vi "Begin.vi"(11 "Image Size":T1=enum."160x120") -> (0 "error out":errorcluster)   [LabVIEW 2012]
doc: "Called before other user functions, this VI is expected to open initial I/O refnums, load in file data, and do all program initialization. Notice that the <B>error out</B> terminal is simply used for data flow. Wiring it to other structures or subVIs ensures that this VI runs first."
uses:
  <vilib>/Rock Robotics/WPI/Camera/WPI_CameraImageSize.ctl
  <vilib>/Rock Robotics/WPI/Camera/WPI_CameraWhite Balance Values.ctl
  <vilib>/Rock Robotics/WPI/Camera/WPI_CameraExposure Values.ctl
  <vilib>/Rock Robotics/WPI/Camera/WPI_CameraFrameRate.ctl
  <vilib>/Rock Robotics/WPI/DriverStation/WPI_DriverStationRobotMode2.ctl
  <vilib>/Rock Robotics/WPI/Joystick/WPI_JoystickDeviceEnum.ctl
  <vilib>/Rock Robotics/SystemInterfaces/DIO/FPGA_DIORelayChannel.ctl
  <vilib>/Rock Robotics/WPI/Relay/WPI_RelayDirection.ctl
  <vilib>/Rock Robotics/SystemInterfaces/DIO/FPGA_DIOPWMChannel.ctl
  <vilib>/Rock Robotics/SystemInterfaces/DIO/FPGA_DIOChannel.ctl
  <vilib>/Rock Robotics/WPI/Solenoid/WPI_SolenoidChannel.ctl
  <vilib>/Rock Robotics/WPI/Relay/WPI_RelayValue.ctl
  <vilib>/Rock Robotics/WPI/SafetyOutput/WPI_SafetyOutputConfigMenu.ctl
  Robot Global Data.vi
  <vilib>/Rock Robotics/WPI/Solenoid/WPI_SolenoidOpenSingle.vi
  <vilib>/Rock Robotics/WPI/MotorControl/WPI_MotorControlOpen Victor.vi
  <vilib>/Rock Robotics/WPI/RobotDrive/WPI_RobotDriveOpen2MotorWithTalon.vi
  <vilib>/Rock Robotics/WPI/Compressor/WPI_CompressorGetSetRefNum.vi
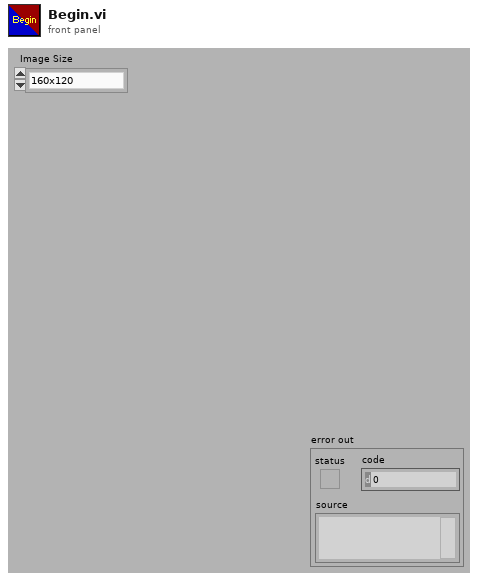
[diagram p1: front panel]
types:
  T1 = typedef "WPI_CameraImageSize.ctl" = enum16{"640x480", "320x240", "160x120"}
  T2 = typedef "FPGA_DIOChannel.ctl" = enum8{"DIO 1", "DIO 2", "DIO 3", "DIO 4", "DIO 5", "DIO 6", "DIO 7", "DIO 8", "DIO 9", "DIO 10", "DIO 11", "DIO 12", "DIO 13", "DIO 14", "Invalid"}
  T3 = typedef "WPI_JoystickDeviceEnum.ctl" = enum16{"USB 1", "USB 2", "USB 3", "USB 4", "Kinect 1", "Kinect 2"}
  T4 = typedef "WPI_SafetyOutputConfigMenu.ctl" = enum16{"Enable", "Disable"}
  T5 = typedef "WPI_SolenoidChannel.ctl" = enum8{"Solenoid 1", "Solenoid 2", "Solenoid 3", "Solenoid 4", "Solenoid 5", "Solenoid 6", "Solenoid 7", "Solenoid 8", "Invalid"}
  T6 = typedef "FPGA_DIOPWMChannel.ctl" = enum8{"PWM 1", "PWM 2", "PWM 3", "PWM 4", "PWM 5", "PWM 6", "PWM 7", "PWM 8", "PWM 9", "PWM 10", "Invalid"}
  T7 = typedef "WPI_RelayValue.ctl" = enum16{"Off", "On", "Forward", "Reverse"}
  T8 = typedef "FPGA_DIORelayChannel.ctl" = enum8{"Relay 1", "Relay 2", "Relay 3", "Relay 4", "Relay 5", "Relay 6", "Relay 7", "Relay 8", "Invalid"}
  T9 = typedef "WPI_RelayDirection.ctl" = enum16{"Both directions", "Forward only", "Reverse only"}
  T10 = typedef "WPI_DriverStationRobotMode2.ctl" = enum16{"Autonomous Disabled", "Autonomous Enabled", "Teleop Disabled", "Teleop Enabled", "Timeout", "Finish", "Test Disabled", "Test Enabled"}
  T11 = typedef "WPI_CameraFrameRate.ctl" = u32
  T12 = typedef "WPI_CameraExposure Values.ctl" = enum16{"Auto", "Flicker-free 50 Hz", "Flicker-free 60 Hz", "Hold current"}
  T13 = typedef "WPI_CameraWhite Balance Values.ctl" = enum16{"Auto", "Fixed indoor", "Fixed outdoor 1", "Fixed outdoor 2", "Fixed fluorescent 1", "Fixed fluorescent 2", "Hold current"}
  T14 = typedef "WPI_MotorControlDeviceRef.ctl" = cluster{"DeviceStatus":errorcluster, "Type":enum16{"PWM", "CAN"}, "PWM":cluster{"Digital Module":T15, "PWM Channel":T6, "DeadBand":T16}, "CAN":cluster{"Device Number":u8, "Control Mode":T17, "Semaphore":T18, "Max Vout":dbl}, "Invert":bool, "TransformRef":T19, "InvTransformRef":T19}
  T15 = typedef "FPGA_TypedefDigitalModule.ctl" = enum16{"Digital Module 1", "Digital Module 2"}
  T16 = typedef "WPI_PWMDeadband.ctl" = cluster{"Name":string, "maxPositivePwm":i32, "minPositivePwm":i32, "centerPwm":i32, "maxNegativePwm":i32, "minNegativePwm":i32, "angularRange":u16}
  T17 = typedef "WPI_CANJaguar_ControlMode.ctl" = enum8{"Percent VBus", "Current", "Speed", "Position", "Voltage"}
  T18 = typedef "Semaphore RefNum" = refnum<k1>
  T19 = typedef "WPI_PWMTransform_ConPane.ctl" = refnum<vi>
  T20 = typedef "WPI_ServoDeviceRef.ctl" = cluster{"DeviceStatus":errorcluster, "Digital Module":T15, "PWM Channel":T6, "DeadBand":T16}
  T21 = typedef "WPI_JoystickDevRef.ctl" = cluster{"Device":T3}
  T22 = typedef "WPI_CameraDevRef.ctl" = cluster{"Camera Address":string, "CameraStatus":errorcluster, "Acquire Image Notifier":refnum<notifier>}
  T23 = typedef "WPI_RobotDriveDevRef.ctl" = cluster{"DevStatus":errorcluster, "Motors[]":T14[], "Square Inputs":bool, "Max Output":dbl, "Isochronous":bool}
  T24 = typedef "WPI_RelayDevRef.ctl" = cluster{"DevStatus":errorcluster, "Relay Channel":T8, "Digital Module":T15, "Relay Direction":T9}
  T25 = typedef "WPI_SolenoidDevRef.ctl" = cluster{"DevStatus":errorcluster, "Solenoid Module":T26, "Forward Solenoid Channel":T5, "Reverse Solenoid Channel":T5}
  T26 = typedef "FPGA_TypedefSolenoidModule.ctl" = enum16{"Solenoid Module 1", "Solenoid Module 2"}
  T27 = typedef "WPI_DigitalInputDevRef.ctl" = cluster{"DevStatus":errorcluster, "DIO Channel":T2, "Digital Module":T15}
  T28 = typedef "WPI_CompressorDevRef.ctl" = cluster{"DevStatus":errorcluster, "DigitalInputDevRef":T27, "RelayDevRef":T24}
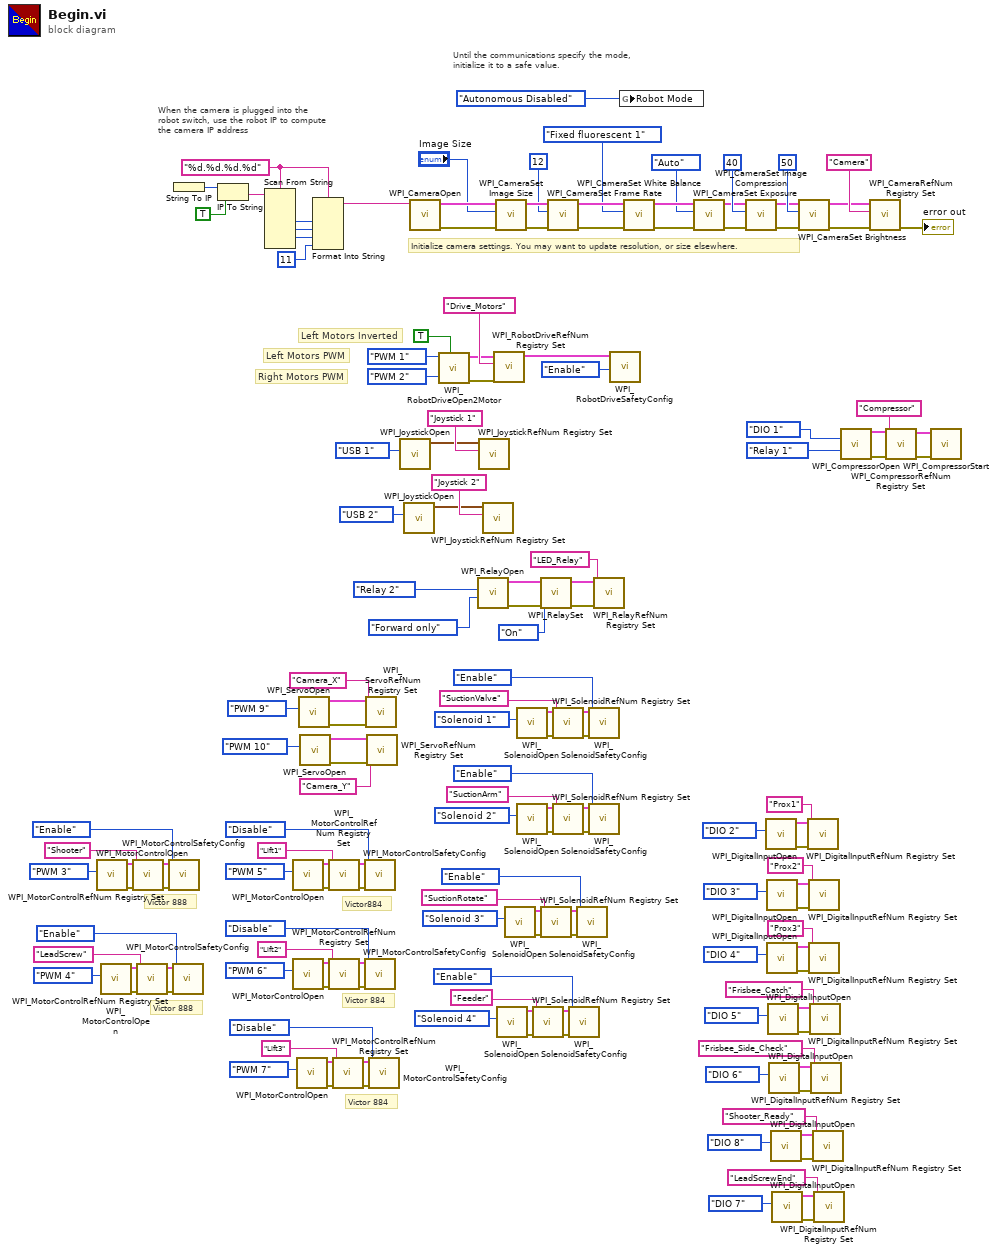
[diagram p0: block diagram]
diagram:
  w131 = "%d.%d.%d.%d" ("format string")
  # "Victor884"
  # "Victor 884"
  # "Victor 884"
  # "Victor 888"
  # "Victor 888"
  # "Right Motors PWM"
  # "Left Motors PWM"
  # "Left Motors Inverted"
  # "Until the communications specify the mode,\ninitialize it to a safe value."
  # "When the camera is plugged into the\nrobot switch, use the robot IP to compute\nthe camera IP address"
  # "Initialize camera settings. You may want to update resolution, or size elsewhere."
  n1 = call-poly <vilib>:"WPI_MotorControlOpen.vi"("PWM Channel"=FPGA_DIOPWMChannel."PWM 3") -> ("error out"=w37:errorcluster, "MotorControlDeviceRef"=w38:T14)  [unwired: 9 in]
  n2 = call-poly <vilib>:"WPI_MotorControlOpen.vi"("PWM Channel"=FPGA_DIOPWMChannel."PWM 4") -> ("error out"=w93:errorcluster, "MotorControlDeviceRef"=w94:T14)  [unwired: 9 in]
  n3 = call <vilib>:"WPI_MotorControlRefNum Registry Set.vi"("error in (no error)"=w37, "refnum name"="Shooter", "MotorControlDevRef"=w38) -> ("error out"=w35:errorcluster, "MotorControlDevRef"=w34:T14)  [unwired: 7 in]
  n4 = call <vilib>:"WPI_MotorControlRefNum Registry Set.vi"("error in (no error)"=w93, "refnum name"="LeadScrew", "MotorControlDevRef"=w94) -> ("error out"=w91:errorcluster, "MotorControlDevRef"=w90:T14)  [unwired: 7 in]
  n5 = call <vilib>:"WPI_MotorControlSafetyConfig.vi"("error in (no error)"=w35, "mode"=WPI_SafetyOutputConfigMenu."Enable", "MotorControlDevRef"=w34) -> ()  [unwired: 7 in, 2 out]
  n6 = call <vilib>:"WPI_MotorControlSafetyConfig.vi"("error in (no error)"=w91, "mode"=WPI_SafetyOutputConfigMenu."Enable", "MotorControlDevRef"=w90) -> ()  [unwired: 7 in, 2 out]
  n7 = String To IP() -> (0:w138:u32)  [unwired: 1 in]
  n8 = IP To String(1:TRUE ("dot notation? (F)"), 2:w138) -> (0:w136:string)
  n9 = Scan From String(format string=w131, input string=w136) -> (output 1=w135:i32, output 2=w134:i32, output 3=w133:i32)  [unwired: 7 in, 3 out]
  n10 = call-poly <vilib>:"WPI_MotorControlOpen.vi"("PWM Channel"=FPGA_DIOPWMChannel."PWM 5") -> ("error out"=w58:errorcluster, "MotorControlDeviceRef"=w59:T14)  [unwired: 9 in]
  n11 = call-poly <vilib>:"WPI_MotorControlOpen.vi"("PWM Channel"=FPGA_DIOPWMChannel."PWM 6") -> ("error out"=w51:errorcluster, "MotorControlDeviceRef"=w52:T14)  [unwired: 9 in]
  n12 = call-poly <vilib>:"WPI_MotorControlOpen.vi"("PWM Channel"=FPGA_DIOPWMChannel."PWM 7") -> ("error out"=w30:errorcluster, "MotorControlDeviceRef"=w31:T14)  [unwired: 9 in]
  n13 = call <vilib>:"WPI_ServoOpen.vi"("PWM Channel"=FPGA_DIOPWMChannel."PWM 9") -> ("error out"=w116:errorcluster, "ServoDeviceRef"=w117:T20)  [unwired: 9 in]
  n14 = call <vilib>:"WPI_ServoOpen.vi"("PWM Channel"=FPGA_DIOPWMChannel."PWM 10") -> ("error out"=w118:errorcluster, "ServoDeviceRef"=w119:T20)  [unwired: 9 in]
  n15 = Format Into String(format string=w131, w135, w134, w133, 11 ("Compression")) -> (resulting string=w127:string)  [unwired: 2 in, 1 out]
  n16 = call <vilib>:"WPI_MotorControlRefNum Registry Set.vi"("error in (no error)"=w58, "refnum name"="Lift1", "MotorControlDevRef"=w59) -> ("error out"=w56:errorcluster, "MotorControlDevRef"=w55:T14)  [unwired: 7 in]
  n17 = call <vilib>:"WPI_MotorControlRefNum Registry Set.vi"("error in (no error)"=w51, "refnum name"="Lift2", "MotorControlDevRef"=w52) -> ("error out"=w49:errorcluster, "MotorControlDevRef"=w48:T14)  [unwired: 7 in]
  n18 = call <vilib>:"WPI_MotorControlRefNum Registry Set.vi"("error in (no error)"=w30, "refnum name"="Lift3", "MotorControlDevRef"=w31) -> ("error out"=w28:errorcluster, "MotorControlDevRef"=w27:T14)  [unwired: 7 in]
  n19 = call <vilib>:"WPI_MotorControlSafetyConfig.vi"("error in (no error)"=w56, "mode"=WPI_SafetyOutputConfigMenu."Disable", "MotorControlDevRef"=w55) -> ()  [unwired: 7 in, 2 out]
  n20 = call <vilib>:"WPI_MotorControlSafetyConfig.vi"("error in (no error)"=w49, "mode"=WPI_SafetyOutputConfigMenu."Disable", "MotorControlDevRef"=w48) -> ()  [unwired: 7 in, 2 out]
  n21 = call <vilib>:"WPI_ServoRefNum Registry Set.vi"("error in (no error)"=w116, "refnum name"="Camera_X", "ServoDeviceRef"=w117) -> ()  [unwired: 7 in, 2 out]
  n22 = call <vilib>:"WPI_ServoRefNum Registry Set.vi"("error in (no error)"=w118, "refnum name"="Camera_Y", "ServoDeviceRef"=w119) -> ()  [unwired: 7 in, 2 out]
  n23 = call <vilib>:"WPI_MotorControlSafetyConfig.vi"("error in (no error)"=w28, "mode"=WPI_SafetyOutputConfigMenu."Disable", "MotorControlDevRef"=w27) -> ()  [unwired: 7 in, 2 out]
  n24 = call <vilib>:"WPI_JoystickOpen.vi"("JoystickDevice"=WPI_JoystickDeviceEnum."USB 1") -> ("JoystickDevRef"=w125:T21)  [unwired: 10 in]
  n25 = call <vilib>:"WPI_JoystickOpen.vi"("JoystickDevice"=WPI_JoystickDeviceEnum."USB 2") -> ("JoystickDevRef"=w6:T21)  [unwired: 10 in]
  n26 = call <vilib>:"WPI_CameraOpen.vi"("Camera Address"=w127) -> ("error out"=w150:errorcluster, "CameraDevRef"=w151:T22)  [unwired: 1 in, 8 out]
  n27 = call-poly <vilib>:"WPI_RobotDriveOpen2Motor.vi"("Left Motor Inverted"=TRUE, "Right Motor"=FPGA_DIOPWMChannel."PWM 2", "Left Motor"=FPGA_DIOPWMChannel."PWM 1") -> ("error out"=w89:errorcluster, "RobotDriveDevRef"=w88:T23)  [unwired: 7 in]
  n28 = call <vilib>:"WPI_RelayOpen.vi"("Relay Direction"=WPI_RelayDirection."Forward only", "Relay Channel"=FPGA_DIORelayChannel."Relay 2") -> ("error out"=w100:errorcluster, "RelayDevRef"=w99:T24)  [unwired: 8 in]
  n29 = call <vilib>:"WPI_JoystickRefNum Registry Set.vi"("refnum name"="Joystick 1", "JoystickDevRef"=w125) -> ()  [unwired: 8 in, 2 out]
  n30 = call <vilib>:"WPI_JoystickRefNum Registry Set.vi"("refnum name"="Joystick 2", "JoystickDevRef"=w6) -> ()  [unwired: 8 in, 2 out]
  n31 = call <vilib>:"WPI_RobotDriveRefNum Registry Set.vi"("error in (no error)"=w89, "refnum name"="Drive_Motors", "RobotDriveDevRef"=w88) -> ("RobotDriveDevRef"=w130:T23)  [unwired: 8 out]
  n32 = call <vilib>:"WPI_CameraSet Image Size.vi"("error in (no error)"=w150, "Image Size"="Image Size", "CameraDevRef"=w151) -> ("error out"=w149:errorcluster, "CameraDevRef Out"=w152:T22)  [unwired: 7 out]
  n33 = call-poly <vilib>:"WPI_SolenoidOpen.vi"("Solenoid Channel"=WPI_SolenoidChannel."Solenoid 4") -> ("error out"=w13:errorcluster, "SolenoidDevRef"=w14:T25)  [unwired: 9 in]
  n34 = call-poly <vilib>:"WPI_SolenoidOpen.vi"("Solenoid Channel"=WPI_SolenoidChannel."Solenoid 3") -> ("error out"=w24:errorcluster, "SolenoidDevRef"=w25:T25)  [unwired: 9 in]
  n35 = call-poly <vilib>:"WPI_SolenoidOpen.vi"("Solenoid Channel"=WPI_SolenoidChannel."Solenoid 1") -> ("error out"=w103:errorcluster, "SolenoidDevRef"=w104:T25)  [unwired: 9 in]
  n36 = call-poly <vilib>:"WPI_SolenoidOpen.vi"("Solenoid Channel"=WPI_SolenoidChannel."Solenoid 2") -> ("error out"=w45:errorcluster, "SolenoidDevRef"=w46:T25)  [unwired: 9 in]
  n37 = call <vilib>:"WPI_SolenoidRefNum Registry Set.vi"("error in (no error)"=w13, "refnum name"="Feeder", "SolenoidDevRef"=w14) -> ("error out"=w10:errorcluster, "SolenoidDevRef"=w9:T25)  [unwired: 7 in]
  n38 = call <vilib>:"WPI_RelaySet.vi"("error in (no error)"=w100, "RelayValue"=WPI_RelayValue."On", "RelayDevRef"=w99) -> ("error out"=w97:errorcluster, "RelayDevRef"=w98:T24)  [unwired: 7 in]
  n39 = call <vilib>:"WPI_SolenoidRefNum Registry Set.vi"("error in (no error)"=w24, "refnum name"="SuctionRotate", "SolenoidDevRef"=w25) -> ("error out"=w21:errorcluster, "SolenoidDevRef"=w20:T25)  [unwired: 7 in]
  n40 = call <vilib>:"WPI_CameraSet Frame Rate.vi"("error in (no error)"=w149, "Frame Rate (fps)"=T11 12, "CameraDevRef"=w152) -> ("error out"=w148:errorcluster, "CameraDevRef Out"=w154:T22)  [unwired: 7 out]
  n41 = call <vilib>:"WPI_SolenoidRefNum Registry Set.vi"("error in (no error)"=w103, "refnum name"="SuctionValve", "SolenoidDevRef"=w104) -> ("error out"=w76:errorcluster, "SolenoidDevRef"=w75:T25)  [unwired: 7 in]
  n42 = call <vilib>:"WPI_SolenoidRefNum Registry Set.vi"("error in (no error)"=w45, "refnum name"="SuctionArm", "SolenoidDevRef"=w46) -> ("error out"=w42:errorcluster, "SolenoidDevRef"=w41:T25)  [unwired: 7 in]
  n43 = call <vilib>:"WPI_SolenoidSafetyConfig.vi"("error in (no error)"=w10, "mode"=WPI_SafetyOutputConfigMenu."Enable", "SolenoidDevRef"=w9) -> ()  [unwired: 7 in, 2 out]
  n44 = call <vilib>:"WPI_SolenoidSafetyConfig.vi"("error in (no error)"=w21, "mode"=WPI_SafetyOutputConfigMenu."Enable", "SolenoidDevRef"=w20) -> ()  [unwired: 7 in, 2 out]
  n45 = call <vilib>:"WPI_SolenoidSafetyConfig.vi"("error in (no error)"=w76, "mode"=WPI_SafetyOutputConfigMenu."Enable", "SolenoidDevRef"=w75) -> ()  [unwired: 7 in, 2 out]
  n46 = call <vilib>:"WPI_SolenoidSafetyConfig.vi"("error in (no error)"=w42, "mode"=WPI_SafetyOutputConfigMenu."Enable", "SolenoidDevRef"=w41) -> ()  [unwired: 7 in, 2 out]
  n47 = call <vilib>:"WPI_RelayRefNum Registry Set.vi"("error in (no error)"=w97, "refnum name"="LED_Relay", "RelayDevRef"=w98) -> ()  [unwired: 7 in, 2 out]
  n48 = call <vilib>:"WPI_RobotDriveSafetyConfig.vi"("mode"=WPI_SafetyOutputConfigMenu."Enable", "RobotDriveDevRef"=w130) -> ()  [unwired: 8 in, 2 out]
  n49 = global write "Robot Global Data.vi" "Robot Mode"(WPI_DriverStationRobotMode2."Autonomous Disabled" ("Robot Mode")) -> ()
  n50 = call <vilib>:"WPI_CameraSet White Balance.vi"("error in (no error)"=w148, "White Balance"=WPI_CameraWhite_Balance_Values."Fixed fluorescent 1", "CameraDevRef"=w154) -> ("error out"=w147:errorcluster, "CameraDevRef Out"=w153:T22)  [unwired: 7 out]
  n51 = call <vilib>:"WPI_CameraSet Exposure.vi"("error in (no error)"=w147, "Exposure"=WPI_CameraExposure_Values."Auto", "CameraDevRef"=w153) -> ("error out"=w146:errorcluster, "CameraDevRef Out"=w156:T22)  [unwired: 7 out]
  n52 = call <vilib>:"WPI_CameraSet Image Compression.vi"("error in (no error)"=w146, "Compression"=40, "CameraDevRef"=w156) -> ("error out"=w145:errorcluster, "CameraDevRef Out"=w155:T22)  [unwired: 7 out]
  n53 = call <vilib>:"WPI_DigitalInputOpen.vi"("DIO Channel"=FPGA_DIOChannel."DIO 2") -> ("error out"=w84:errorcluster, "DigitalInputDevRef"=w83:T27)  [unwired: 9 in]
  n54 = call <vilib>:"WPI_DigitalInputOpen.vi"("DIO Channel"=FPGA_DIOChannel."DIO 3") -> ("error out"=w80:errorcluster, "DigitalInputDevRef"=w79:T27)  [unwired: 9 in]
  n55 = call <vilib>:"WPI_DigitalInputOpen.vi"("DIO Channel"=FPGA_DIOChannel."DIO 4") -> ("error out"=w72:errorcluster, "DigitalInputDevRef"=w71:T27)  [unwired: 9 in]
  n56 = call <vilib>:"WPI_DigitalInputOpen.vi"("DIO Channel"=FPGA_DIOChannel."DIO 5") -> ("error out"=w68:errorcluster, "DigitalInputDevRef"=w67:T27)  [unwired: 9 in]
  n57 = call <vilib>:"WPI_DigitalInputOpen.vi"("DIO Channel"=FPGA_DIOChannel."DIO 6") -> ("error out"=w64:errorcluster, "DigitalInputDevRef"=w63:T27)  [unwired: 9 in]
  n58 = call <vilib>:"WPI_DigitalInputOpen.vi"("DIO Channel"=FPGA_DIOChannel."DIO 8") -> ("error out"=w18:errorcluster, "DigitalInputDevRef"=w17:T27)  [unwired: 9 in]
  n59 = call <vilib>:"WPI_DigitalInputOpen.vi"("DIO Channel"=FPGA_DIOChannel."DIO 7") -> ("error out"=w4:errorcluster, "DigitalInputDevRef"=w3:T27)  [unwired: 9 in]
  n60 = call <vilib>:"WPI_CameraSet Brightness.vi"("error in (no error)"=w145, "Brightness"=50, "CameraDevRef"=w155) -> ("error out"=w143:errorcluster, "CameraDevRef Out"=w144:T22)  [unwired: 7 out]
  n61 = call <vilib>:"WPI_DigitalInputRefNum Registry Set.vi"("error in (no error)"=w84, "refnum name"="Prox1", "DigitalInputDevRef"=w83) -> ()  [unwired: 7 in, 2 out]
  n62 = call <vilib>:"WPI_DigitalInputRefNum Registry Set.vi"("error in (no error)"=w80, "refnum name"="Prox2", "DigitalInputDevRef"=w79) -> ()  [unwired: 7 in, 2 out]
  n63 = call <vilib>:"WPI_DigitalInputRefNum Registry Set.vi"("error in (no error)"=w72, "refnum name"="Prox3", "DigitalInputDevRef"=w71) -> ()  [unwired: 7 in, 2 out]
  n64 = call <vilib>:"WPI_DigitalInputRefNum Registry Set.vi"("error in (no error)"=w68, "refnum name"="Frisbee_Catch", "DigitalInputDevRef"=w67) -> ()  [unwired: 7 in, 2 out]
  n65 = call <vilib>:"WPI_DigitalInputRefNum Registry Set.vi"("error in (no error)"=w64, "refnum name"="Frisbee_Side_Check", "DigitalInputDevRef"=w63) -> ()  [unwired: 7 in, 2 out]
  n66 = call <vilib>:"WPI_DigitalInputRefNum Registry Set.vi"("error in (no error)"=w18, "refnum name"="Shooter_Ready", "DigitalInputDevRef"=w17) -> ()  [unwired: 7 in, 2 out]
  n67 = call <vilib>:"WPI_DigitalInputRefNum Registry Set.vi"("error in (no error)"=w4, "refnum name"="LeadScrewEnd", "DigitalInputDevRef"=w3) -> ()  [unwired: 7 in, 2 out]
  n68 = call <vilib>:"WPI_CompressorOpen.vi"("Pressure Switch DIO Channel"=FPGA_DIOChannel."DIO 1", "Relay Channel"=FPGA_DIORelayChannel."Relay 1") -> ("CompressorDevRef"=w108:T28, "error out"=w109:errorcluster)  [unwired: 12 in]
  n69 = call <vilib>:"WPI_CameraRefNum Registry Set.vi"("error in (no error)"=w143, "refnum name"="Camera", "CameraDevRef"=w144) -> ("error out"=→"error out":errorcluster)  [unwired: 8 out]
  n70 = call <vilib>:"WPI_CompressorRefNum Registry Set.vi"("error in (no error)"=w109, "refnum name"="Compressor", "CompressorDevRef"=w108) -> ("error out"=w106:errorcluster, "CompressorDevRef"=w105:T28)  [unwired: 7 in]
  n71 = call <vilib>:"WPI_CompressorStart.vi"("error in (no error)"=w106, "CompressorDevRef"=w105) -> ()  [unwired: 8 in, 2 out]
